vi "Acquire Callback1.vi"() -> ()   [LabVIEW 2019]
doc: "Generates sample waveforms according to the signal type in the HW Config input."
uses:
  Settings/System Running Settings.ctl
  HardwareAdapter/Support/Hardware Configuration.ctl
  HardwareAdapter/Support/Camera Configuration.ctl
  C:/RM21-MMicrosopeSource/HardwareAdapter/Camera/Dependencies/PVCamNET.dll
  HardwareAdapter/Camera/Dependencies/PVCamNET.dll
  <vilib>/vision/Image Controls.llb/IMAQ Image.ctl
  C:/RM21-MMicrosopeSource/HardwareAdapter/Lasers/Dependencies/Oxxius_Boxx.dll
  HardwareAdapter/Lasers/Dependencies/Oxxius_Boxx.dll
  Logging/Logging Configuration.ctl
  Controls/DeviceStatusCtl.ctl
  Controls/CallBack Refs.ctl
  DataQueuesAndNotifier.ctl
  Logging/Logging.lvlib
  Settings/Settings.lvlib
panel:
  in  "EnQueue?":bool=TRUE
  in  "DataQueuesAndNotifier":T1
  in  "FrameIndex":i32
  out "Config Out":T2 {"Hardware Configuration"."Lasers Configuration"."SettingValues"."785 Power" format="%.1f"; "Hardware Configuration"."Lasers Configuration"."SettingValues"."647 Power" format="%.1f"; "Hardware Configuration"."Lasers Configuration"."SettingValues"."561 Power" format="%.1f"}
  in  "Config In":T2 {"Hardware Configuration"."Lasers Configuration"."SettingValues"."785 Power" format="%.1f"; "Hardware Configuration"."Lasers Configuration"."SettingValues"."647 Power" format="%.1f"; "Hardware Configuration"."Lasers Configuration"."SettingValues"."561 Power" format="%.1f"}
  in  "error in (no error)":errorcluster
  out "error out":errorcluster
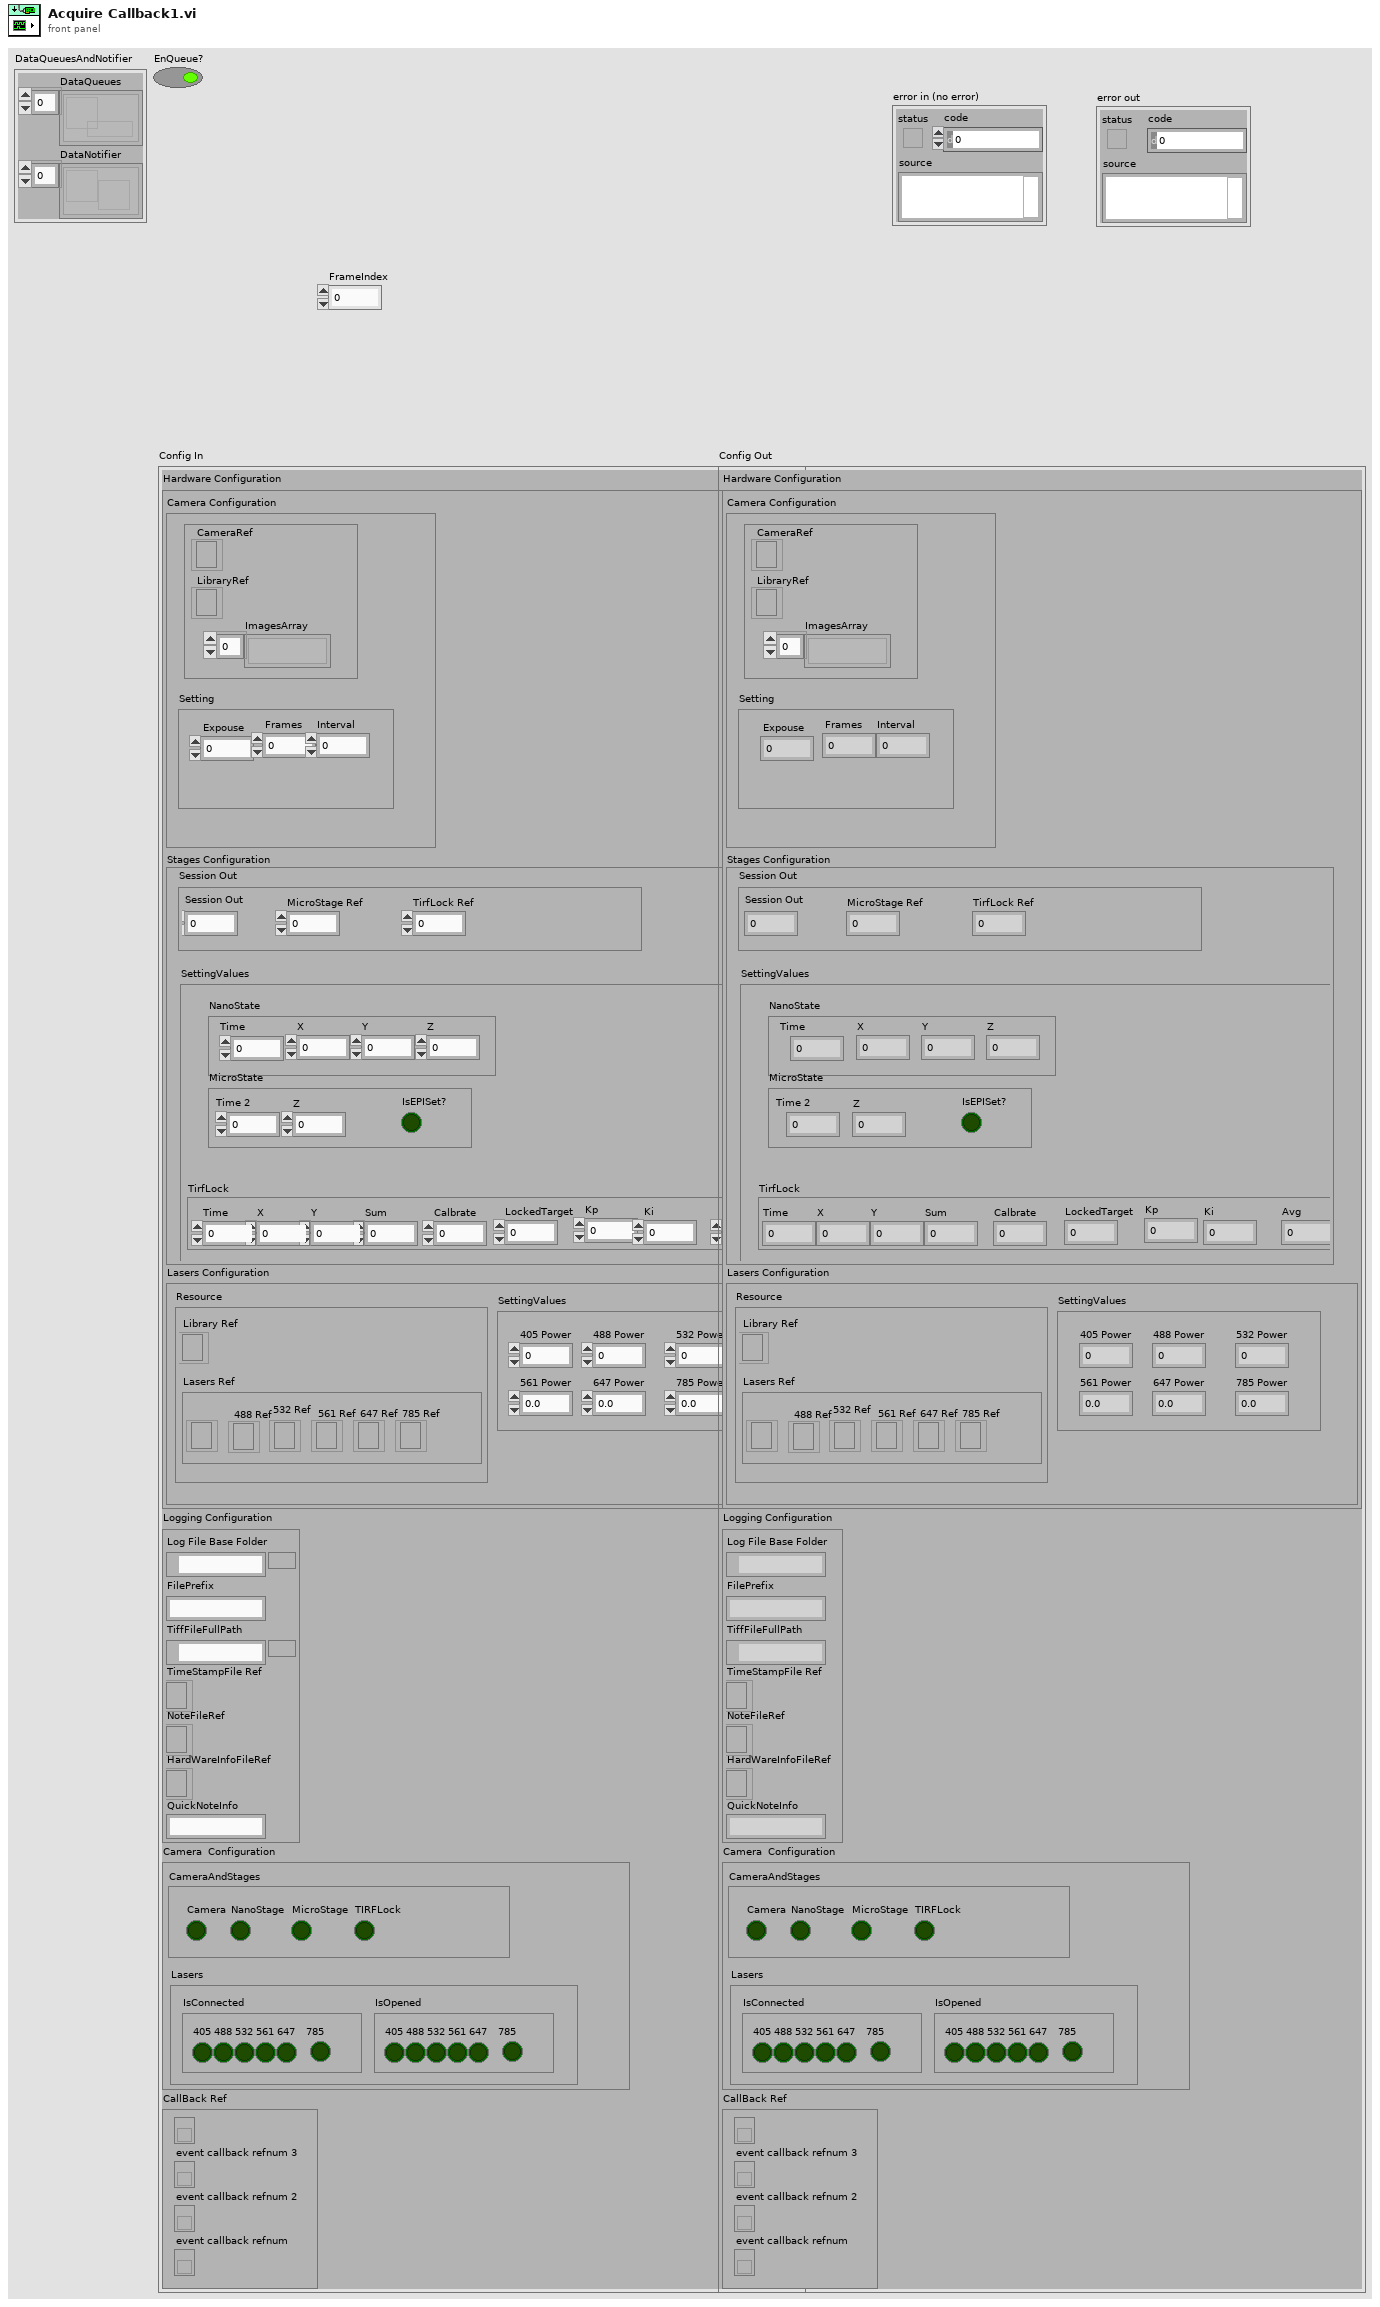
[diagram p1: front panel]
types:
  T1 = typedef "DataQueuesAndNotifier.ctl" = cluster{"DataQueues":refnum<queue>[], "DataNotifier":refnum<notifier>[]}
  T2 = typedef "Settings.lvlib/System Running Settings.ctl" = cluster{"Hardware Configuration":T3, "Logging Configuration":T6, "HardWare Status":cluster{"CameraAndStages":T7, "Lasers":cluster{"IsConnected":cluster{"405":bool, "488":bool, "532":bool, "561":bool, "647":bool, "785":bool}, "IsOpened":cluster{"405":bool, "488":bool, "532":bool, "561":bool, "647":bool, "785":bool}}}, "CallBack Ref":T8}
  T3 = typedef "Hardware Configuration.ctl" = cluster{"Camera Configuration":T4, "Stages Configuration":cluster{"Resource":cluster{"NanoStage Ref":i32, "MicroStage Ref":i32, "TirfLock Ref":i32}, "SettingValues":cluster{"NanoState":cluster{"Time":dbl, "X":dbl, "Y":dbl, "Z":dbl}, "MicroState":cluster{"Time 2":dbl, "Z":dbl, "IsEPISet?":bool}, "TirfLock":cluster{"Time":dbl, "X":dbl, "Y":dbl, "Sum":dbl, "Calbrate":dbl, "LockedTarget":dbl, "Kp":dbl, "Ki":dbl, "Avg":dbl}}}, "Lasers Configuration":cluster{"SettingValues":cluster{"405 Power":sgl, "488 Power":sgl, "532 Power":sgl, "561 Power":sgl, "647 Power":sgl, "785 Power":sgl}, "Resource":cluster{"Library Ref":refnum<k24>, "Lasers Ref":cluster{"405 Ref":refnum<k24>, "488 Ref":refnum<k24>, "532 Ref":refnum<k24>, "561 Ref":refnum<k24>, "647 Ref":refnum<k24>, "785 Ref":refnum<k24>}}}}
  T4 = typedef "Camera Configuration.ctl" = cluster{"Setting":cluster{"Expouse":dbl, "Frames":dbl, "Interval":dbl}, "Resource":cluster{"CameraRef":refnum<k24>, "LibraryRef":refnum<k24>, "ImagesArray":T5[]}}
  T5 = typedef "IMAQ Image.ctl" = refnum<image>
  T6 = typedef "Logging.lvlib/Logging Configuration.ctl" = cluster{"Log File Base Folder":path, "FilePrefix":string, "TiffFileFullPath":path, "TimeStampFile Ref":refnum<file>, "NoteFileRef":refnum<file>, "HardWareInfoFileRef":refnum<file>, "QuickNoteInfo":string}
  T7 = typedef "DeviceStatusCtl.ctl" = cluster{"Camera":bool, "NanoStage":bool, "MicroStage":bool, "TIRFLock":bool}
  T8 = typedef "CallBack Refs.ctl" = cluster{"event callback refnum":refnum<k27>, "event callback refnum 2":refnum<k27>, "event callback refnum 3":refnum<k27>, "event callback refnum 4":refnum<k27>}
  T9 = typedef "Image MatadataCtl.ctl" = cluster{"TimeStamp(Acq)":dbl, "Image":T5, "Histogram":u32[], "MeanValue":dbl, "Min":u32, "Max":u32, "FrameIndex":dbl, "TimeStamp(Album)":dbl}
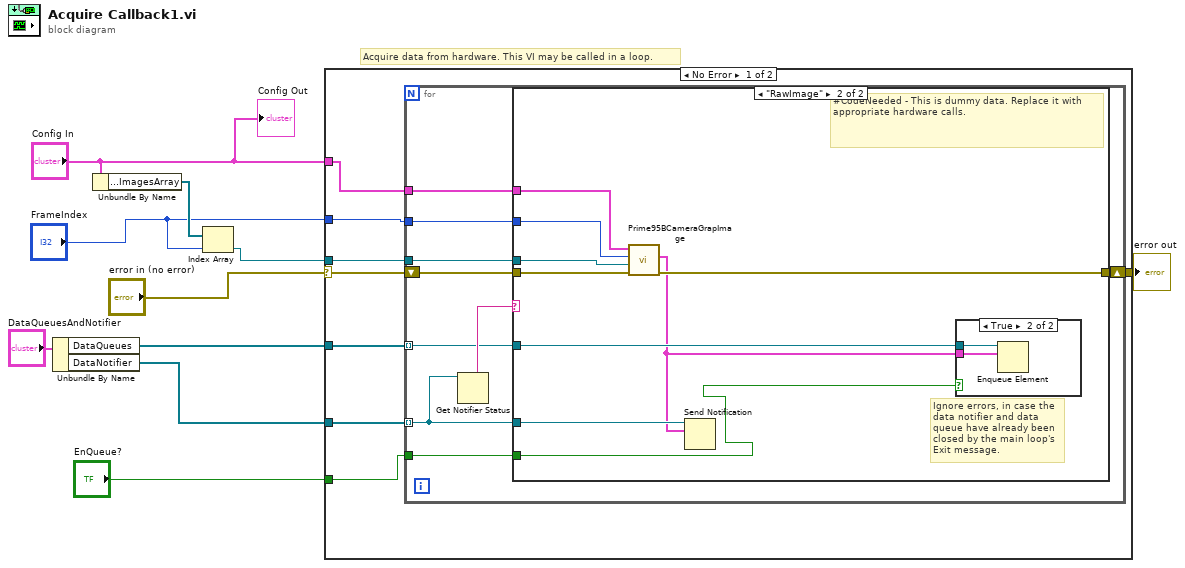
[diagram p0: block diagram]
diagram:
  # "Acquire data from hardware. This VI may be called in a loop."
  n1 = Unbundle By Name("DataQueuesAndNotifier") -> ("DataQueues"=w6:refnum<queue>[], "DataNotifier"=w7:refnum<notifier>[])
  n2 = Unbundle By Name("Config In") -> ("Hardware Configuration.Camera Configuration.Resource.ImagesArray"=w3:T5[])
  n3 = Index Array(array=w3, index="FrameIndex") -> (element=w1:T5)
  n4 = case shown="No Error" "error in (no error)" {
    selector: "error in (no error)" -> [w18 w40]
    tunnel: [w17 w40] -> w9
    tunnel: w7 -> [w15 _]
    tunnel: "Config In" -> [w16 _]
    tunnel: "FrameIndex" -> [w14 _]
    tunnel: w6 -> [w13 _]
    tunnel: "EnQueue?" -> [w12 _]
    tunnel: w1 -> [w11 _]
    frame No Error {
      n5 = for {
        tunnel: w16 -> [w25]
        shift-right: [w26] -> w17
        shift-left: w18 -> [w27]
        tunnel: w15 -> [w24] mode=indexing
        tunnel: w14 -> [w22]
        tunnel: w13 -> [w21] mode=indexing
        tunnel: w12 -> [w20]
        tunnel: w11 -> [w19]
        n6 = Get Notifier Status(notifier=w24) -> (notifier name=w23:string)  [unwired: 1 in, 4 out]
        n7 = case shown="\"RawImage\"" w23 {
          tunnel: w27 -> [w28 w37]
          tunnel: [w28 w36] -> w26
          tunnel: w25 -> [_ w35]
          tunnel: w24 -> [_ w34]
          tunnel: w22 -> [_ w33]
          tunnel: w21 -> [_ w32]
          tunnel: w20 -> [_ w30]
          tunnel: w19 -> [_ w29]
          frame "False", Default {
          }
          frame "RawImage" {
            # "Ignore errors, in case the data notifier and data queue have already been closed by the main loop's Exit message."
            # "#CodeNeeded - This is dummy data. Replace it with appropriate hardware calls."
            n8 = call "Prime95BCameraGrapImage.vi"("error in (no error)"=w37, "New Image"=w29, "FrameIndex"=w33, "Config In"=w35) -> ("error out"=w36:errorcluster, "RawImage"=w31:T9)  [unwired: 4 in, 1 out]
            n9 = Send Notification(notification=w31, notifier=w34) -> ()  [unwired: 1 in, 2 out]
            n10 = case shown="True" w30 {
              tunnel: w32 -> [_ w39]
              tunnel: w31 -> [_ w38]
              frame False {
              }
              frame True {
                n11 = Enqueue Element(queue=w39, element=w38) -> ()  [unwired: 2 in, 3 out]
              }
            }
          }
        }
      }
    }
    frame Error {
    }
  }
  "error out" <- w9
  "Config Out" <- "Config In"
